vi "Queue_LV2.vi"(0 "Name":string, 7 "State":string, 11 "Error in":errorcluster, 13 "Queue Operations":T1) -> (4 "Dequeue State":string, 15 "Error out":errorcluster)   [LabVIEW 2020, in "ADC_MultiChannel.lvlib"]
doc: "This VI is a Queue Driver. Here all the queue operations are made into separate cases."
uses:
  ADC_MultiChannel.lvlib
  Typedefs/Queue_Operations.ctl
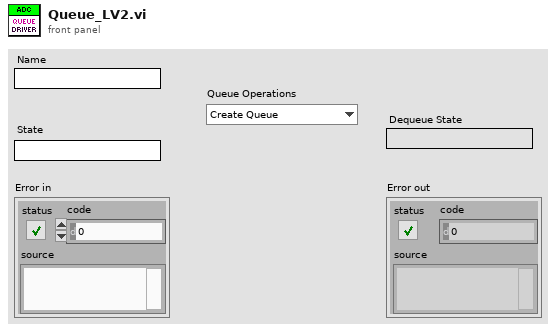
[diagram p1: front panel]
types:
  T1 = typedef "ADC_MultiChannel.lvlib/Queue_Operations.ctl" = enum16{"Create Queue", "Enqueue element", "Dequeue", "Flush Queue", "Close Queue"}
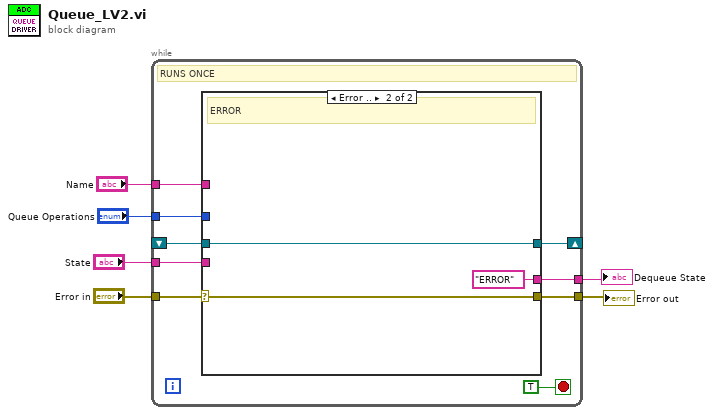
[diagram p0: block diagram]
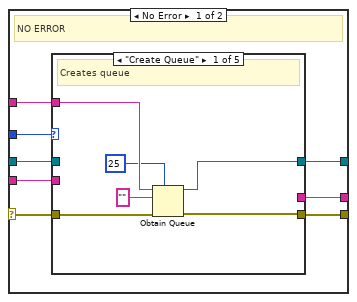
[diagram p2: hidden frame]
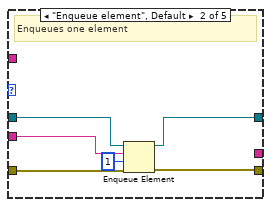
[diagram p3: hidden frame]
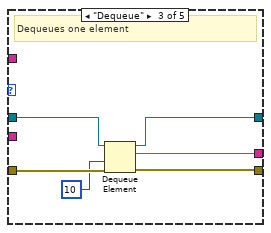
[diagram p4: hidden frame]
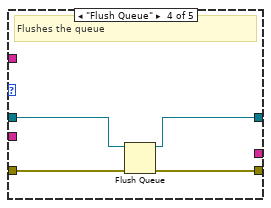
[diagram p5: hidden frame]
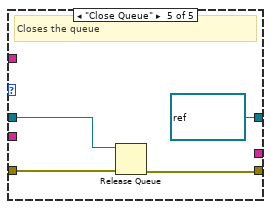
[diagram p6: hidden frame]
diagram:
  n1 = while {
    tunnel: "Error in" -> [w15]
    tunnel: [w14] -> w5
    tunnel: "Queue Operations" -> [w13]
    tunnel: "Name" -> [w12]
    shift-right: [w10] -> _
    shift-left: _ -> [w11]
    tunnel: "State" -> [w9]
    tunnel: [w8] -> w1
    stop <- TRUE stop-if-true
    # "RUNS ONCE"
    n2 = case shown="Error .." w15 {
      selector: w15 -> [w23 w52]
      tunnel: [w22 w52] -> w14
      tunnel: w13 -> [w21 _]
      tunnel: w12 -> [w20 _]
      tunnel: w11 -> [w19 w51]
      tunnel: [w18 w51] -> w10
      tunnel: w9 -> [w17 _]
      tunnel: [w16 "ERROR"] -> w8
      frame No Error {
        # "NO ERROR"
        n3 = case shown="\"Create Queue\"" w21 {
          tunnel: [w28 w34 w40 w45 w48] -> w22
          tunnel: w23 -> [w29 w35 w41 w44 w49]
          tunnel: w20 -> [w27 _ _ _ _]
          tunnel: w19 -> [_ w33 w38 w43 w47]
          tunnel: [w25 w32 w39 w42 refnum<queue> refnum ("queue out")] -> w18
          tunnel: w17 -> [_ w31 _ _ _]
          tunnel: [_ _ w36 _ _] -> w16
          frame "Create Queue" {
            # "Creates queue"
            n4 = Obtain Queue(max queue size (-1, unlimited)=25, name (unnamed)=w27, element data type="", error in (no error)=w29) -> (queue out=w25:refnum<queue>, error out=w28:errorcluster)  [unwired: 1 in, 1 out]
          }
          frame "Enqueue element", Default {
            # "Enqueues one element"
            n5 = Enqueue Element(queue=w33, element=w31, timeout in ms (-1)=1, error in (no error)=w35) -> (queue out=w32:refnum<queue>, error out=w34:errorcluster)  [unwired: 1 out]
          }
          frame "Dequeue" {
            # "Dequeues one element"
            n6 = Dequeue Element(queue=w38, timeout in ms (-1)=10, error in (no error)=w41) -> (queue out=w39:refnum<queue>, element=w36:string, error out=w40:errorcluster)  [unwired: 1 out]
          }
          frame "Flush Queue" {
            # "Flushes the queue"
            n7 = Flush Queue(queue=w43, error in (no error)=w44) -> (queue out=w42:refnum<queue>, error out=w45:errorcluster)  [unwired: 1 out]
          }
          frame "Close Queue" {
            # "Closes the queue"
            n8 = Release Queue(queue=w47, error in (no error)=w49) -> (error out=w48:errorcluster)  [unwired: 1 in, 2 out]
          }
        }
      }
      frame Error {
        # "ERROR"
      }
    }
  }
  "Error out" <- w5
  "Dequeue State" <- w1
